vi "ReadVoltageFromLockinAndConverttToTemperature.vi"(8 "error in 2":errorcluster) -> (0 "error out 2":errorcluster, 3 "Temperature":dbl=200.0 format="%.2f")   [LabVIEW 2010]
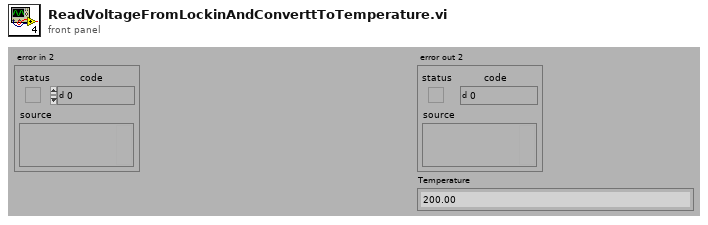
[diagram p1: front panel]
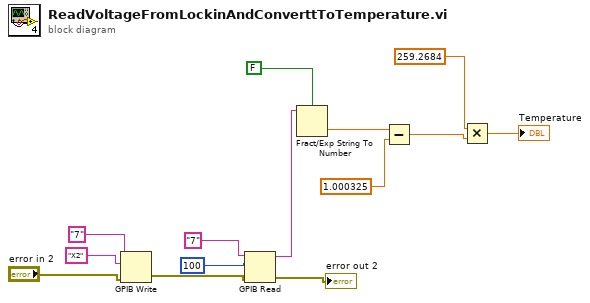
[diagram p0: block diagram]
diagram:
  n1 = GPIB Write(0:"7", 1:"X2", 3:"error in 2") -> (6:w11:errorcluster)  [unwired: 2 in, 1 out]
  n2 = GPIB Read(0:"7", 1:100, 3:w11) -> (5:w8:string, 7:→"error out 2":errorcluster)  [unwired: 2 in, 1 out]
  n3 = Fract/Exp String To Number(use system decimal point (T)=FALSE, string=w8) -> (number=w5:dbl)  [unwired: 2 in, 1 out]
  n4 = Subtract(x=w5, y=1.000325) -> (x-y=w3:dbl)
  n5 = Multiply(x=259.2684, y=w3) -> (x*y=→"Temperature":dbl)
